vi "CurrentPSUSettings.vi"() -> ()   [LabVIEW 2017]
panel:
  in  "Tr":dbl
  in  "Immediate Voltage set":dbl
  in  "Immediate Current set":dbl
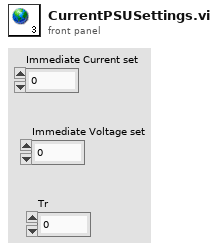
[diagram p1: front panel]
diagram:
